vi "Create Datasets.vi"() -> ()   [LabVIEW 2020]
uses:
  ctl/Connection Information.ctl
  <vilib>/addons/database/Connection.llb/Conn ObjectReference.ctl
  <vilib>/addons/database/Connection.llb/DB Tools Open Connec (String).vi
  <vilib>/addons/database/Connection.llb/DB Tools Open Connec (Path).vi
  <vilib>/addons/database/Connection.llb/Conn Execute.vi
  <vilib>/addons/database/Recordset.llb/Rec Fetch Recordset Data (R).vi
  <vilib>/addons/database/Recordset.llb/Rec Destroy - Connection.vi
  <vilib>/addons/database/_DB Variant To Data/Database Variant To Data.xnode
  <vilib>/addons/database/NI_Database_API.lvlib
panel:
  in  "Back Square":bool
  in  "Save Data Set":bool
  in  "Build Query":bool
  out "Query":string
  in  "Records":string[](tree)
  in  "Move Right":bool
  in  "Move Left":bool
  out "error out":errorcluster
  out "data":string[][](array[string])
  out "Get Values on Tree":bool
  in  "Database Tree":string[](tree)
  in  "error in (no error)":errorcluster
  in  "Connect Button":bool
  in  "stop":bool
  in  "Connection Information":T1
  in  "Data Sources":string(combo)
  # "SELECT DATA SOURCE"
  # "SELECT COLUMN"
  # "CREATE DATA SETS"
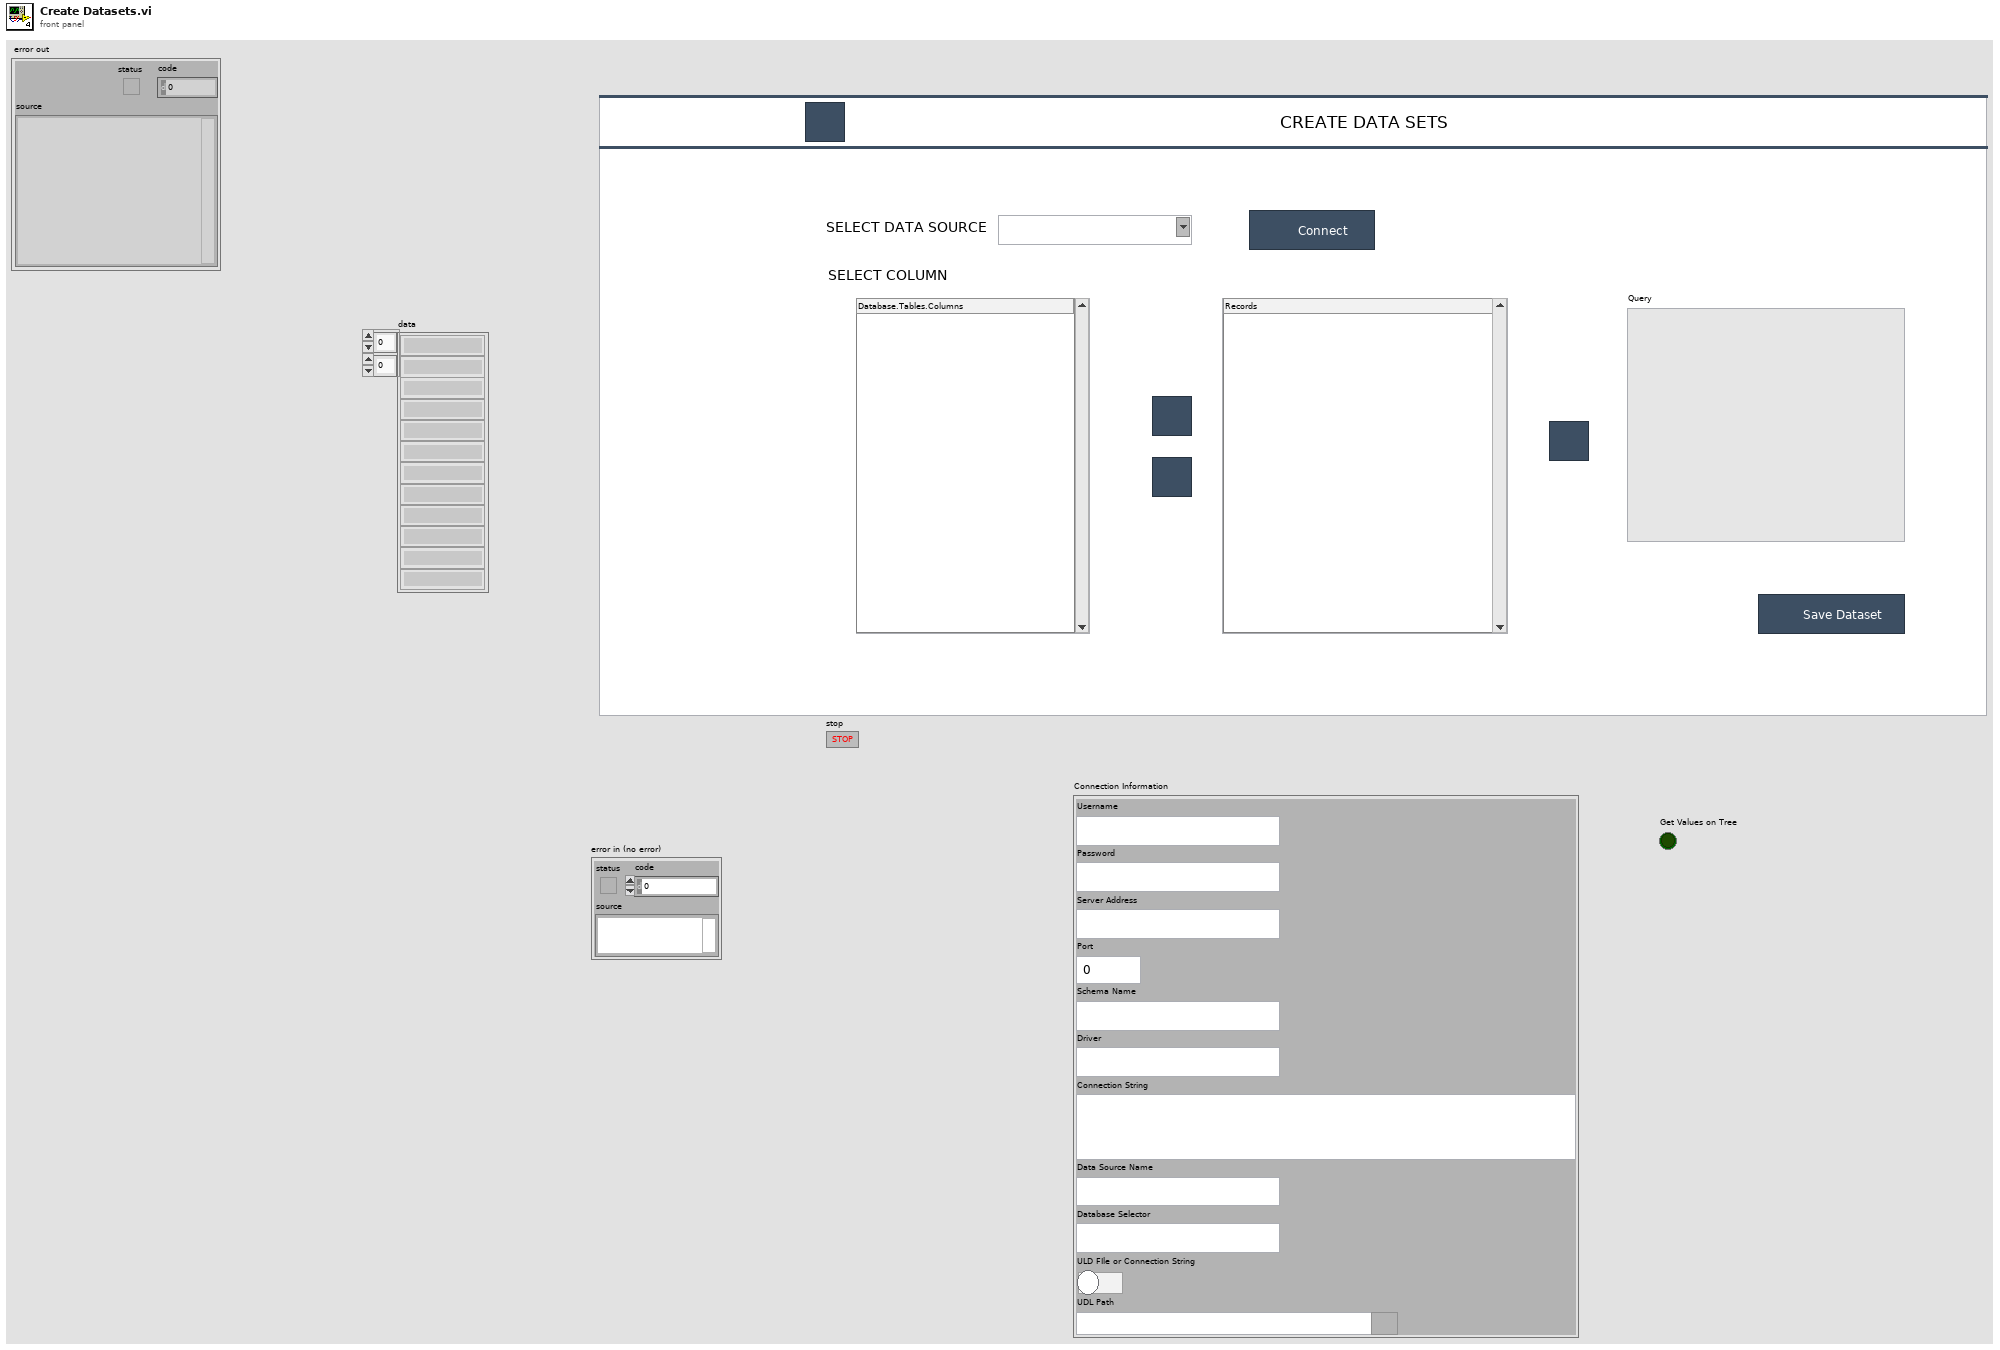
[diagram p1: front panel]
types:
  T1 = typedef "Connection Information.ctl" = cluster{"Username":string, "Password":string, "Server Address":string, "Port":u32, "Schema Name":string, "Driver":string, "Connection String":string, "Data Source Name":string, "Database Selector":string, "ULD FIle or Connection String":bool, "UDL Path":path}
  T2 = typedef "Config Cluster.ctl" = cluster{"MYSQL":cluster{"SHOW DATABASE":string, "SHOW TABLES":string, "SHOW COLUMNS":string}, "SQL Server":cluster{"SHOW DATABASE":string, "SHOW TABLES":string, "SHOW COLUMNS":string}}
  T3 = cluster{"Left Cell String":string, "Child Text":string[], "Child Tag":string, "Item Indent":i32, "Child Only?":bool, "Glyph Index":i32}
  T4 = typedef "NI_Database_API.lvlib/Conn ObjectReference.ctl" = refnum<k1>
  T5 = typedef "NI_Database_API.lvlib/Rec ObjectReference.ctl" = refnum<k1>
  T6 = cluster{"Left Cell String":string, "Child Text":string[], "Child Tag":string, "Item Indent":i32, "Child Only?":bool, "Glyph Index":i32}[]
  T7 = cluster{"Query":string, "DB Type":string, "Data Source name":string}
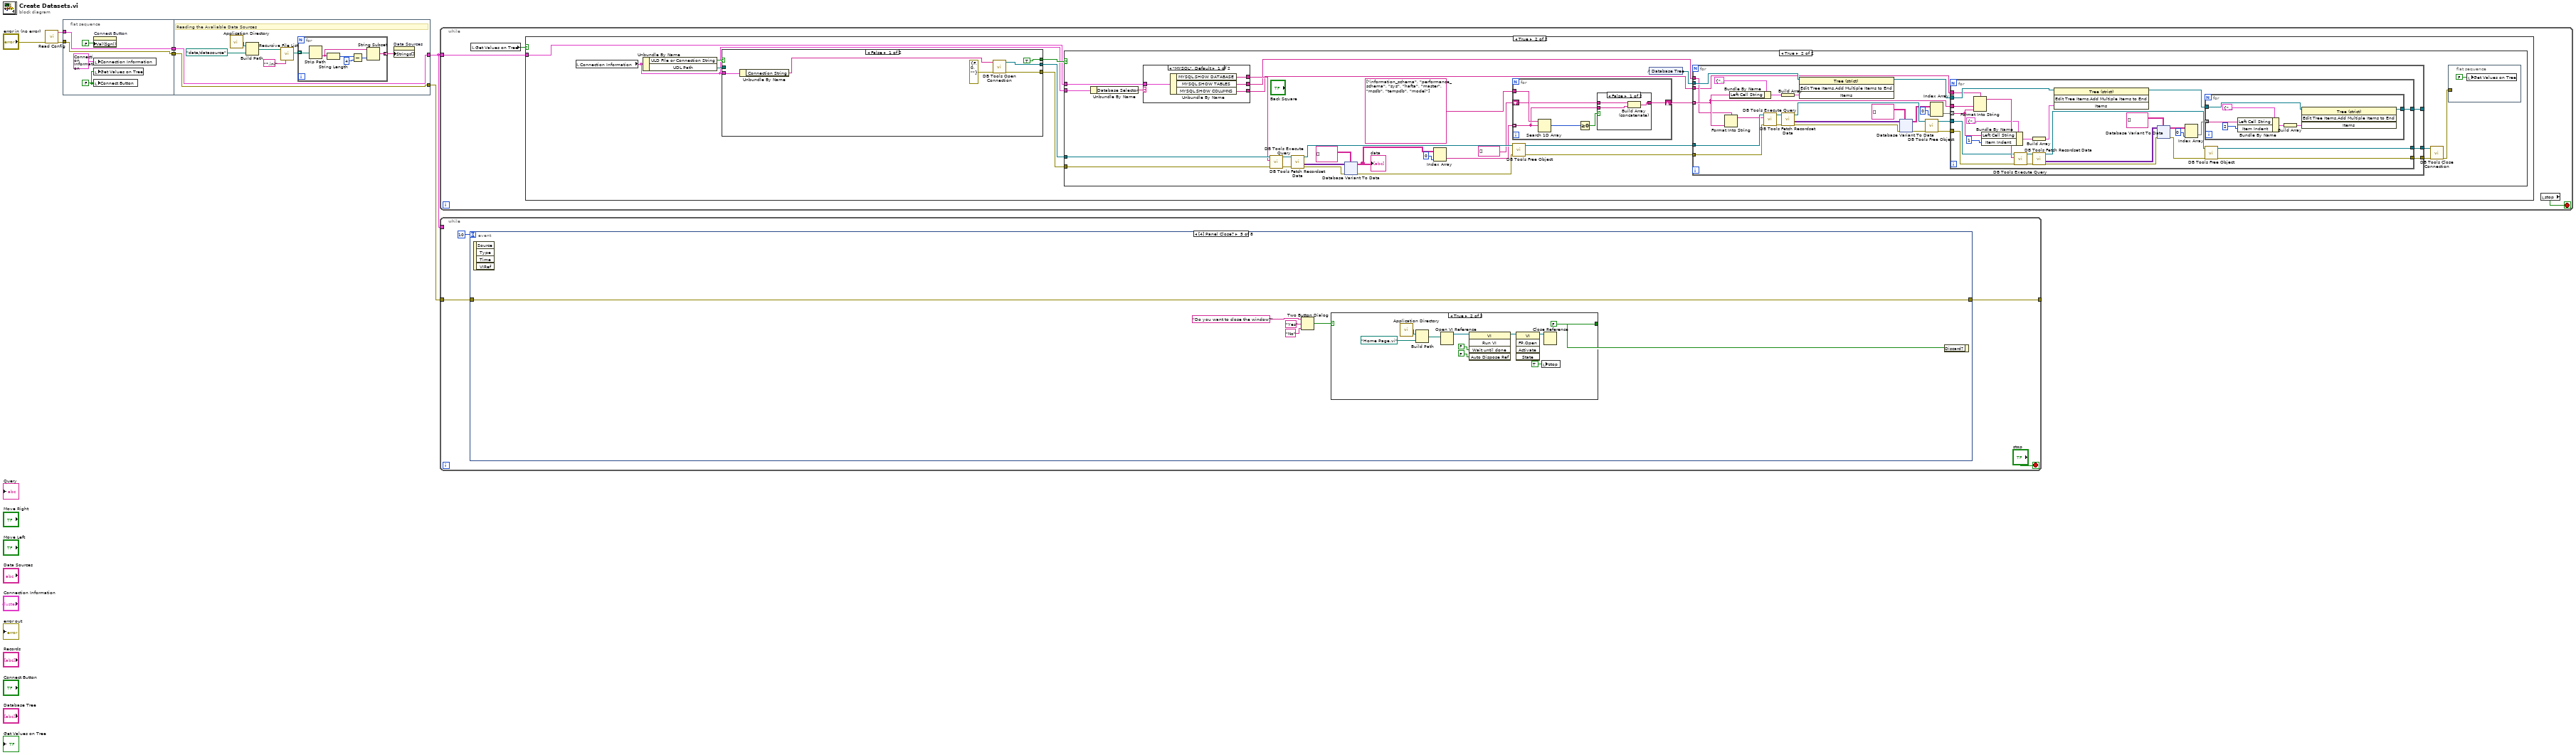
[diagram p0: block diagram]
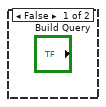
[diagram p2: hidden frame]
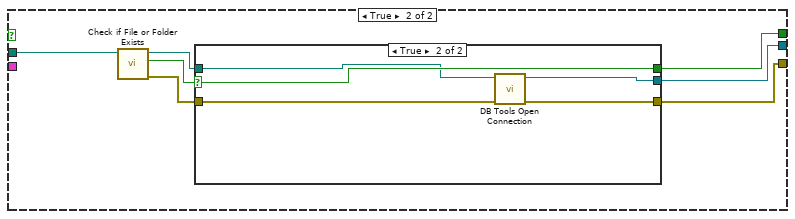
[diagram p3: hidden frame]
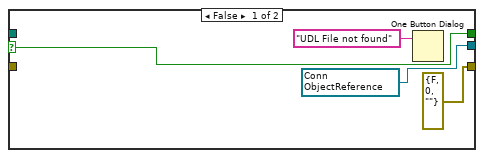
[diagram p4: hidden frame]
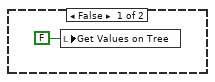
[diagram p5: hidden frame]
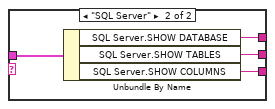
[diagram p6: hidden frame]
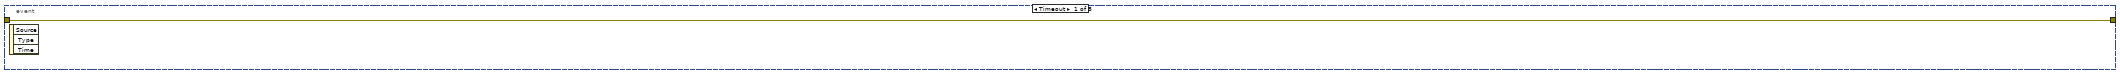
[diagram p8: hidden frame]
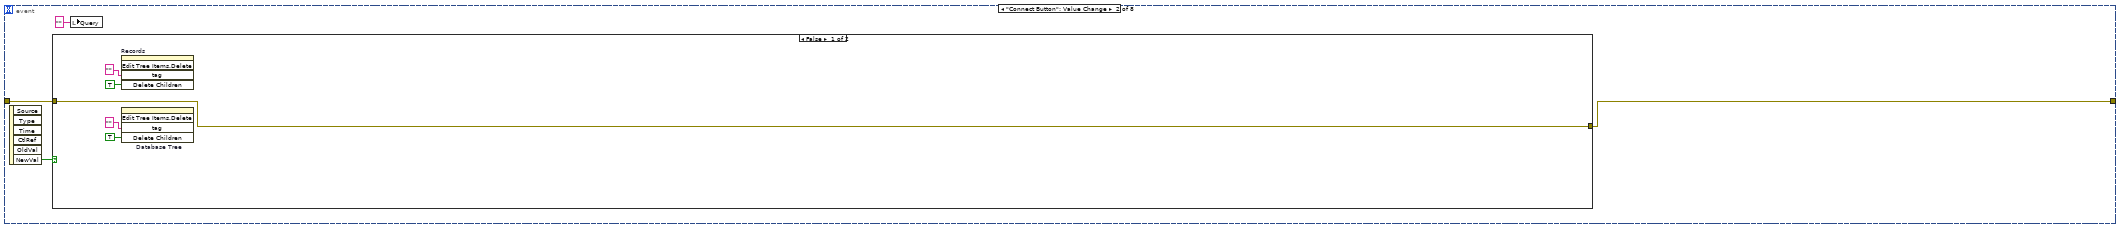
[diagram p9: hidden frame]
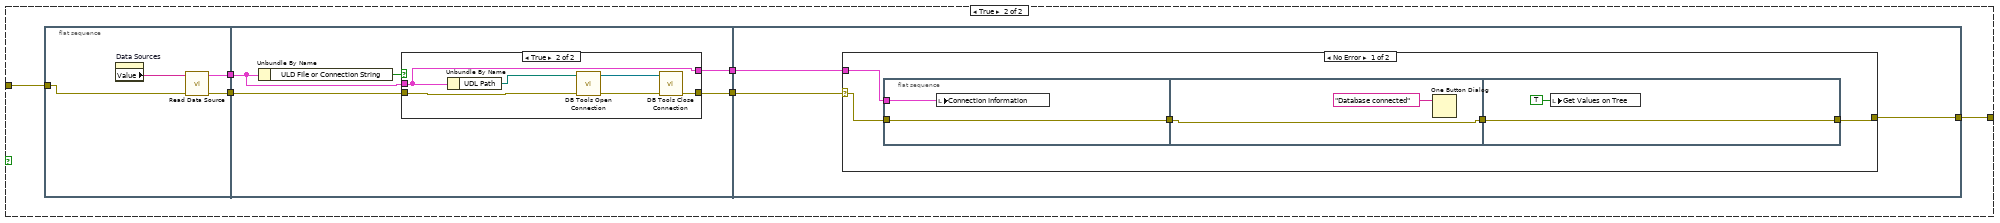
[diagram p10: hidden frame]
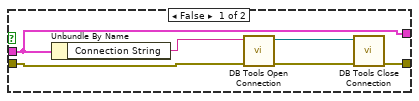
[diagram p11: hidden frame]
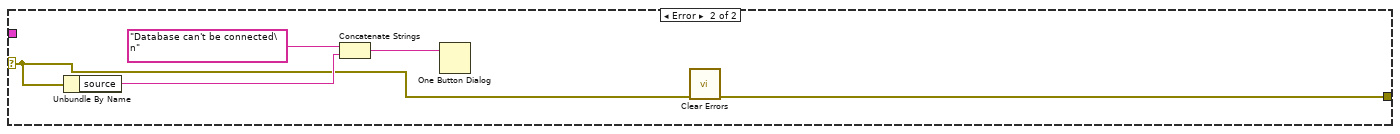
[diagram p12: hidden frame]
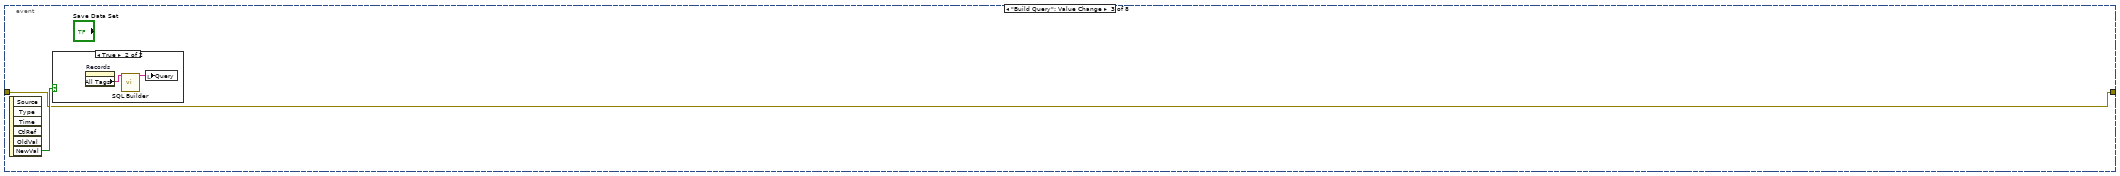
[diagram p13: hidden frame]
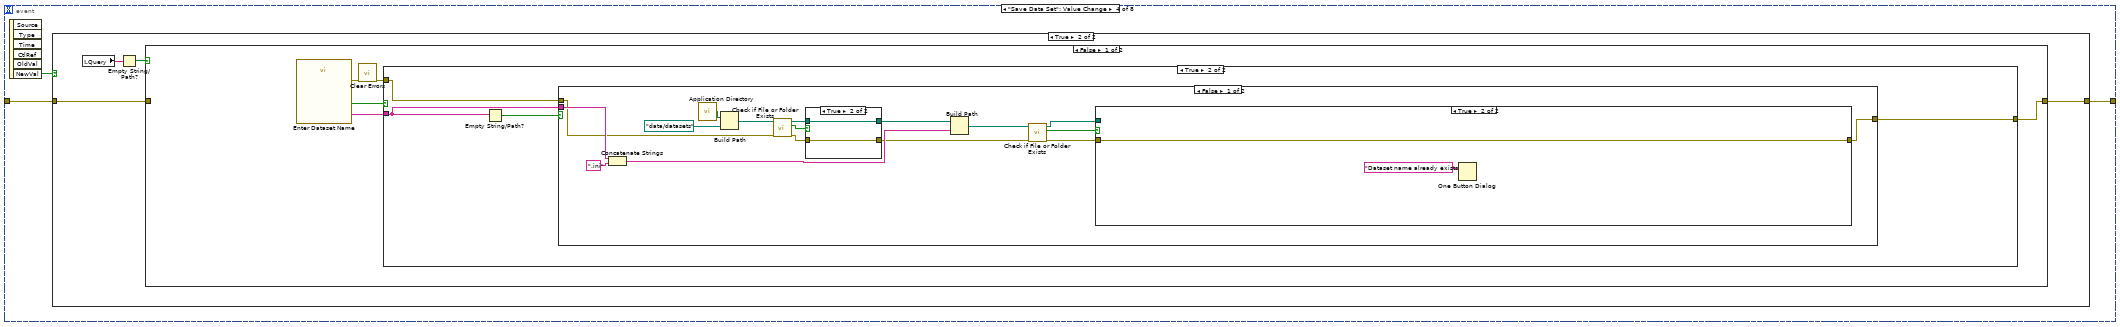
[diagram p15: hidden frame]
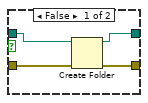
[diagram p18: hidden frame]
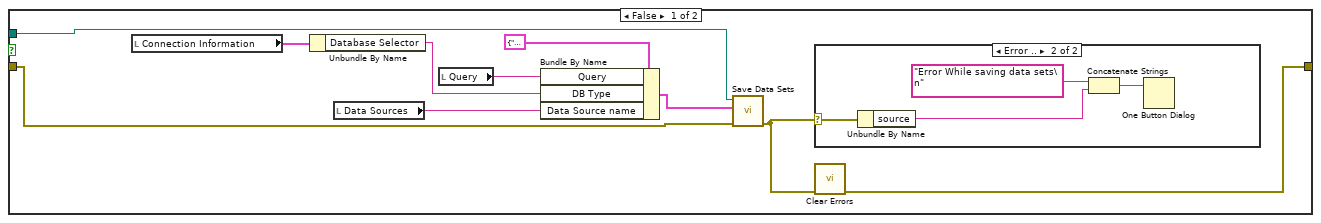
[diagram p19: hidden frame]
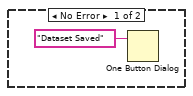
[diagram p20: hidden frame]
diagram:
  n1 = call "Read Config.vi"("error in (no error)"="error in (no error)") -> ("error out"=w1:errorcluster, "Config"=w4:T2)  [unwired: 9 in]
  n2 = flat-sequence {
    tunnel: w1 -> [w12]
    tunnel: [w12] -> w6
    tunnel: [w8] -> w5
    tunnel: w4 -> [w8]
    tunnel: [w20] -> w7
    tunnel: w6 -> [w20]
    tunnel: [w13] -> w3
    tunnel: w5 -> [w13]
    frame #0 {
      w10 = FALSE ("Get Values on Tree")
      n3 = property on="Connect Button" class="Bool (strict)"("Val(Sgnl)"=FALSE ("Value (Signaling)")) -> ()  [unwired: 2 in, 2 out]
      n4 = local write "Connection Information"(T1 {"Username"="", "Password"="", "Server Address"="", "Port"=0, "Schema Name"="", "Driver"="", "Connection String"="", "Data Source Name"="", "Database Selector"="", "ULD FIle or Connection String"=FALSE, "UDL Path"=path ""} ("Connection Information")) -> ()
      n5 = local write "Get Values on Tree"(w10) -> ()
      n6 = local write "Connect Button"(w10) -> ()
    }
    frame #1 {
      # "Reading the Avaliable Data Sources"
      n7 = call <vilib>:"Application Directory.vi"() -> ("Application Directory"=w19:path)
      n8 = Build Path(base path=w19, name or relative path=path "data/datasource") -> (appended path=w17:path)
      n9 = call <vilib>:"Recursive File List.vi"("pattern"="*.ini", "Folder Path"=w17) -> ("All Files in Dir"=w15:path[])  [unwired: 5 in, 4 out]
      n10 = for {
        tunnel: w15 -> [w26] mode=indexing
        tunnel: [w23] -> w14 mode=indexing
        n11 = Strip Path(path=w26) -> (name=w25:string)  [unwired: 1 out]
        n12 = String Length(string=w25) -> (length=w24:i32)
        n13 = Subtract(x=w24, y=4) -> (x-y=w22:i32)
        n14 = String Subset(string=w25, length (rest)=w22) -> (substring=w23:string)  [unwired: 1 in]
      }
      n15 = property on="Data Sources" class="CmbBox"("Strings[]"=w14) -> ()  [unwired: 2 in, 2 out]
    }
  }
  n16 = while {
    tunnel: w3 -> [w28]
    stop <- w29 stop-if-true
    n17 = local read "Get Values on Tree"() -> (w27:bool)
    n18 = case shown="True" w27 {
      tunnel: w28 -> [_ w30]
      frame False {
      }
      frame True {
        n19 = local read "Connection Information"() -> (w31:T1)
        n20 = Unbundle By Name(w31) -> ("ULD FIle or Connection String"=w36:bool, "UDL Path"=w35:path)
        n21 = case shown="False" w36 {
          tunnel: w35 -> [_ w49]
          tunnel: [TRUE ("file or folder exists?") w47] -> w34
          tunnel: [w40 w43] -> w33
          tunnel: [w39 w44] -> w32
          tunnel: w31 -> [w38 _]
          frame False {
            n22 = Unbundle By Name(w38) -> ("Connection String"=w37:string)
            n23 = call-poly <vilib>:"DB Tools Open Connection.vi"("error in (no error)"=errorcluster {"status"=FALSE, "code"=0, "source"=""} ("error out"), "connection information"=w37) -> ("error out"=w40:errorcluster, "connection reference"=w39:T4)  [unwired: 6 in]
          }
          frame True {
            n24 = call <vilib>:"Check if File or Folder Exists.vi"("path"=w49) -> ("error out"=w45:errorcluster, "file or folder exists?"=w48:bool, "dup path"=w46:path)  [unwired: 8 in]
            n25 = case shown="True" w48 {
              selector: w48 -> [w52 w58]
              tunnel: [w52 w58] -> w47
              tunnel: w46 -> [_ w57]
              tunnel: w45 -> [_ w56]
              tunnel: [w51 w55] -> w44
              tunnel: [errorcluster {"status"=FALSE, "code"=0, "source"=""} ("error out") w54] -> w43
              frame False {
                w51 = T4 refnum items=["Connection"] ("connection reference")
                n26 = One Button Dialog(message="UDL File not found") -> ()  [unwired: 1 in, 1 out]
              }
              frame True {
                n27 = call-poly <vilib>:"DB Tools Open Connection.vi"("error in (no error)"=w56, "connection information"=w57) -> ("error out"=w54:errorcluster, "connection reference"=w55:T4)  [unwired: 6 in]
              }
            }
          }
        }
        n28 = case shown="True" w34 {
          tunnel: w31 -> [_ w66]
          tunnel: w33 -> [_ w68]
          tunnel: w32 -> [_ w67]
          tunnel: w30 -> [_ w63]
          frame False {
            n29 = local write "Get Values on Tree"(FALSE ("Get Values on Tree")) -> ()
          }
          frame True {
            n30 = Unbundle By Name(w66) -> ("Database Selector"=w65:string)
            n31 = case shown="\"MYSQL\", Default" w65 {
              tunnel: [w90 w94] -> w64
              tunnel: w63 -> [w91 w95]
              tunnel: [w89 w93] -> w62
              tunnel: [w88 w92] -> w61
              frame "MYSQL", Default {
                n32 = Unbundle By Name(w91) -> ("MYSQL.SHOW DATABASE"=w90:string, "MYSQL.SHOW TABLES"=w89:string, "MYSQL.SHOW COLUMNS"=w88:string)
              }
              frame "SQL Server" {
                n33 = Unbundle By Name(w95) -> ("SQL Server.SHOW DATABASE"=w94:string, "SQL Server.SHOW TABLES"=w93:string, "SQL Server.SHOW COLUMNS"=w92:string)
              }
            }
            n34 = call-poly <vilib>:"DB Tools Execute Query.vi"("error in (no error)"=w68, "SQL query"=w64, "connection reference"=w67) -> ("error out"=w85:errorcluster, "recordset reference"=w86:T5)  [unwired: 5 in]
            n35 = call-poly <vilib>:"DB Tools Fetch Recordset Data.vi"("error in (no error)"=w85, "recordset reference"=w86) -> ("error out"=w81:errorcluster, "recordset data"=w83:variant[][], "recordset reference out"=w84:T5)  [unwired: 3 in]
            n36 = xnode "Database Variant To Data"("database variant"=w83, "error in (no error)"=w81, "type"=string[][] []) -> ("data"=w79:string[][], "error out"=w80:errorcluster)
            "data" <- w79
            n37 = Index Array(array=w79, index (col)=0 ("disabled index (col)")) -> (element=w71:string[])  [unwired: 1 in]
            n38 = for {
              tunnel: w71 -> [w96] mode=indexing
              shift-right: [w98] -> w70
              shift-left: string[] [] -> [w97]
              tunnel: string[] ["information_schema", "performance_schema", "sys", "hafta", "master", "msdb", "tempdb", "model"] -> [w101]
              n39 = Search 1D Array(1D array=w101, element=w96) -> (index of element=w100:i32)  [unwired: 1 in]
              n40 = Greater Or Equal To 0?(x=w100) -> (x >= 0?=w99:bool)
              n41 = case shown="False" w99 {
                tunnel: [w102 w105] -> w98
                tunnel: w97 -> [w103 w105]
                tunnel: w96 -> [w104 _]
                frame False {
                  n42 = Build Array (concatenate)(w103, w104) -> (w102:string[])
                }
                frame True {
                }
              }
            }
            n43 = call-poly <vilib>:"DB Tools Free Object.vi"("error in (no error)"=w80, "recordset reference"=w84) -> ("error out"=w76:errorcluster, "connection reference"=w77:T4)  [unwired: 8 in]
            n44 = control-ref of="Database Tree"() -> (w69:refnum<vi>)
            n45 = for {
              tunnel: w77 -> [w130]
              tunnel: w76 -> [w129]
              tunnel: w69 -> [w131]
              tunnel: w70 -> [w109] mode=indexing
              tunnel: [w115] -> w75
              tunnel: [w114] -> w74
              tunnel: [w108] -> _
              tunnel: w62 -> [w107]
              tunnel: w61 -> [w106]
              n46 = Format Into String(format string=w107, w109) -> (resulting string=w128:string)  [unwired: 2 in, 1 out]
              n47 = Bundle By Name(cluster=T3 {"Left Cell String"="", "Child Text"=[], "Child Tag"="", "Item Indent"=0, "Child Only?"=FALSE, "Glyph Index"=0} ("Item"), "Left Cell String"=w109) -> (w112:T3)
              n48 = call-poly <vilib>:"DB Tools Execute Query.vi"("error in (no error)"=w129, "SQL query"=w128, "connection reference"=w130) -> ("error out"=w126:errorcluster, "recordset reference"=w127:T5)  [unwired: 5 in]
              n49 = Build Array(w112) -> (w111:T6)
              n50 = call-poly <vilib>:"DB Tools Fetch Recordset Data.vi"("error in (no error)"=w126, "recordset reference"=w127) -> ("error out"=w122:errorcluster, "recordset data"=w123:variant[][], "recordset reference out"=w125:T5)  [unwired: 3 in]
              n51 = invoke on="Invoke Node" class="Tree (strict)" method="Edit Tree Items.Add Multiple Items to End"(reference=w131, "Items"=w111) -> (reference out=w110:refnum<vi>)  [unwired: 2 in, 3 out]
              n52 = xnode "Database Variant To Data"("database variant"=w123, "error in (no error)"=w122, "type"=string[][] []) -> ("data"=w120:string[][], "error out"=w121:errorcluster)
              n53 = call-poly <vilib>:"DB Tools Free Object.vi"("error in (no error)"=w121, "recordset reference"=w125) -> ("error out"=w116:errorcluster, "connection reference"=w117:T4)  [unwired: 8 in]
              n54 = Index Array(array=w120, index (col)=0 ("disabled index (col)")) -> (element=w118:string[])  [unwired: 1 in]
              n55 = for {
                tunnel: w118 -> [w177] mode=indexing
                tunnel: w117 -> [w190]
                tunnel: w116 -> [w189]
                tunnel: [w188] -> w115
                tunnel: [w187] -> w114
                tunnel: w110 -> [w181]
                tunnel: w109 -> [w178]
                tunnel: [w179] -> w108
                tunnel: w106 -> [w176]
                n56 = Format Into String(format string=w176, w178, w177) -> (resulting string=w191:string)  [unwired: 2 in, 1 out]
                n57 = Bundle By Name(cluster=T3 {"Left Cell String"="", "Child Text"=[], "Child Tag"="", "Item Indent"=0, "Child Only?"=FALSE, "Glyph Index"=0} ("Item"), "Left Cell String"=w177, "Item Indent"=1) -> (w186:T3)
                n58 = call-poly <vilib>:"DB Tools Execute Query.vi"("error in (no error)"=w189, "SQL query"=w191, "connection reference"=w190) -> ("error out"=w193:errorcluster, "recordset reference"=w192:T5)  [unwired: 5 in]
                n59 = Build Array(w186) -> (w184:T6)
                n60 = call-poly <vilib>:"DB Tools Fetch Recordset Data.vi"("error in (no error)"=w193, "recordset reference"=w192) -> ("error out"=w197:errorcluster, "recordset data"=w196:variant[][], "recordset reference out"=w194:T5)  [unwired: 3 in]
                n61 = invoke on="Invoke Node" class="Tree (strict)" method="Edit Tree Items.Add Multiple Items to End"(reference=w181, "Items"=w184) -> (reference out=w180:refnum<vi>)  [unwired: 2 in, 3 out]
                n62 = xnode "Database Variant To Data"("database variant"=w196, "error in (no error)"=w197, "type"=string[][] []) -> ("data"=w199:string[][], "error out"=w198:errorcluster)
                n63 = Index Array(array=w199, index (col)=0 ("disabled index (col)")) -> (element=w182:string[])  [unwired: 1 in]
                n64 = for {
                  tunnel: w182 -> [w203] mode=indexing
                  tunnel: w180 -> [w202]
                  tunnel: [w201] -> w179
                  n65 = Bundle By Name(cluster=T3 {"Left Cell String"="", "Child Text"=[], "Child Tag"="", "Item Indent"=0, "Child Only?"=FALSE, "Glyph Index"=0} ("Item"), "Left Cell String"=w203, "Item Indent"=2) -> (w204:T3)
                  n66 = Build Array(w204) -> (w206:T6)
                  n67 = invoke on="Invoke Node" class="Tree (strict)" method="Edit Tree Items.Add Multiple Items to End"(reference=w202, "Items"=w206) -> (reference out=w201:refnum<vi>)  [unwired: 2 in, 3 out]
                }
                n68 = call-poly <vilib>:"DB Tools Free Object.vi"("error in (no error)"=w198, "recordset reference"=w194) -> ("error out"=w188:errorcluster, "connection reference"=w187:T4)  [unwired: 8 in]
              }
            }
            n69 = call <vilib>:"DB Tools Close Connection.vi"("error in (no error)"=w75, "connection reference"=w74) -> ("error out"=w60:errorcluster)  [unwired: 5 in]
            n70 = flat-sequence {
              tunnel: w60 -> [_]
              frame #0 {
                n71 = local write "Get Values on Tree"(FALSE ("Get Values on Tree")) -> ()
              }
            }
          }
        }
      }
    }
    n72 = local read "stop"() -> (w29:bool)
  }
  n73 = while {
    tunnel: w7 -> [w297]
    tunnel: w3 -> [_]
    tunnel: [w296] -> _
    stop <- "stop" stop-if-true
    n74 = event shown="[4] Panel Close?" {
      selector: _ -> [_ _ _ _ _ _ _ _]
      dyn-events: _ -> [_ _ _ _ _ _ _ _]
      timeout: 10 -> [_ _ _ _ _ _ _ _]
      tunnel: w297 -> [w300 w303 w356 w360 w424 _ w453 w515]
      tunnel: [w300 w302 w356 w361 w424 _ w453 w515] -> w296
      event Timeout {
        n75 = event-data() -> ()  [unwired: 1 in, 3 out]
      }
      event "Connect Button": Value Change {
        n76 = event-data() -> ("NewVal"=w304:bool)  [unwired: 1 in, 5 out]
        n77 = case shown="False" w304 {
          tunnel: w303 -> [w309 w312]
          tunnel: [w309 w311] -> w302
          frame False {
            n78 = invoke on="Records" class="Tree (strict)" method="Edit Tree Items.Delete"("tag"="" ("Tag"), "Delete Children"=TRUE ("Delete Children?")) -> ()  [unwired: 3 in, 5 out]
            n79 = invoke on="Database Tree" class="Tree (strict)" method="Edit Tree Items.Delete"("tag"="" ("Tag"), "Delete Children"=TRUE ("Delete Children?")) -> ()  [unwired: 3 in, 5 out]
          }
          frame True {
            n80 = flat-sequence {
              tunnel: [w318] -> w315
              tunnel: [w317] -> w314
              tunnel: w312 -> [w316]
              tunnel: w315 -> [w324]
              tunnel: w314 -> [w321]
              tunnel: [w323] -> w313
              tunnel: [w320] -> w310
              tunnel: w313 -> [w339]
              tunnel: [w337] -> w311
              tunnel: w310 -> [w338]
              frame #0 {
                n81 = property on="Data Sources" class="CmbBox"() -> ("Value"=w319:string)  [unwired: 2 in, 2 out]
                n82 = call "Read Data Source.vi"("error in (no error)"=w316, "Data Source Name"=w319) -> ("error out"=w318:errorcluster, "Connection Information"=w317:T1)  [unwired: 8 in]
              }
              frame #1 {
                n83 = Unbundle By Name(w321) -> ("ULD FIle or Connection String"=w322:bool)
                n84 = case shown="True" w322 {
                  tunnel: w324 -> [w327 w334]
                  tunnel: [w326 w333] -> w323
                  tunnel: w321 -> [w325 w331]
                  tunnel: [w325 w331] -> w320
                  frame False {
                    n85 = Unbundle By Name(w325) -> ("Connection String"=w328:string)
                    n86 = call-poly <vilib>:"DB Tools Open Connection.vi"("error in (no error)"=w327, "connection information"=w328) -> ("error out"=w330:errorcluster, "connection reference"=w329:T4)  [unwired: 6 in]
                    n87 = call <vilib>:"DB Tools Close Connection.vi"("error in (no error)"=w330, "connection reference"=w329) -> ("error out"=w326:errorcluster)  [unwired: 5 in]
                  }
                  frame True {
                    n88 = Unbundle By Name(w331) -> ("UDL Path"=w332:path)
                    n89 = call-poly <vilib>:"DB Tools Open Connection.vi"("error in (no error)"=w334, "connection information"=w332) -> ("error out"=w336:errorcluster, "connection reference"=w335:T4)  [unwired: 6 in]
                    n90 = call <vilib>:"DB Tools Close Connection.vi"("error in (no error)"=w336, "connection reference"=w335) -> ("error out"=w333:errorcluster)  [unwired: 5 in]
                  }
                }
              }
              frame #2 {
                n91 = case shown="No Error" w339 {
                  selector: w339 -> [w340 w352]
                  tunnel: w338 -> [w344 _]
                  tunnel: [w343 w351] -> w337
                  frame No Error {
                    n92 = flat-sequence {
                      tunnel: w344 -> [w346]
                      tunnel: [w345] -> w341
                      tunnel: w340 -> [w345]
                      tunnel: [w347] -> w342
                      tunnel: w341 -> [w347]
                      tunnel: [w349] -> w343
                      tunnel: w342 -> [w349]
                      frame #0 {
                        n93 = local write "Connection Information"(w346) -> ()
                      }
                      frame #1 {
                        n94 = One Button Dialog(message="Database connected") -> ()  [unwired: 1 in, 1 out]
                      }
                      frame #2 {
                        n95 = local write "Get Values on Tree"(TRUE ("Get Values on Tree")) -> ()
                      }
                    }
                  }
                  frame Error {
                    n96 = Unbundle By Name(w352) -> ("source"=w354:string)
                    n97 = Concatenate Strings("Database can't be connected\n" ("message"), w354) -> (w353:string)
                    n98 = One Button Dialog(message=w353) -> ()  [unwired: 1 in, 1 out]
                    n99 = call <vilib>:"Clear Errors.vi"("error in (no error)"=w352) -> ("error out"=w351:errorcluster)  [unwired: 5 in, 1 out]
                  }
                }
              }
            }
          }
        }
        n100 = local write "Query"("" ("Query")) -> ()
      }
      event "Build Query": Value Change {
        n101 = event-data() -> ("NewVal"=w357:bool)  [unwired: 1 in, 5 out]
        n102 = case shown="True" w357 {
          frame False {
          }
          frame True {
            n103 = property on="Records" class="Tree (strict)"() -> ("All Tags"=w358:string[])  [unwired: 2 in, 2 out]
            n104 = call "SQL Builder.vi"("SELECTED COLUMNS"=w358) -> ("Built Query"=w359:string)  [unwired: 10 in]
            n105 = local write "Query"(w359) -> ()
          }
        }
      }
      event "Save Data Set": Value Change {
        n106 = event-data() -> ("NewVal"=w362:bool)  [unwired: 1 in, 5 out]
        n107 = case shown="True" w362 {
          tunnel: [w363 w365] -> w361
          tunnel: w360 -> [w363 w364]
          frame False {
          }
          frame True {
            n108 = local read "Query"() -> (w367:string)
            n109 = Empty String/Path?(string/path=w367) -> (empty?=w366:bool)
            n110 = case shown="False" w366 {
              tunnel: [w368 w421] -> w365
              tunnel: w364 -> [_ w421]
              frame False {
                n111 = call "Enter Dataset Name"() -> ("Dataset Name"=w369:string, "OK"=w372:bool, "error out"=w371:errorcluster)  [unwired: 17 in]
                n112 = call <vilib>:"Clear Errors.vi"("error in (no error)"=w371) -> ("error out"=w370:errorcluster)  [unwired: 5 in, 1 out]
                n113 = case shown="True" w372 {
                  tunnel: w370 -> [w373 w375]
                  tunnel: w369 -> [_ w376]
                  tunnel: [w373 w374] -> w368
                  frame False {
                  }
                  frame True {
                    n114 = Empty String/Path?(string/path=w376) -> (empty?=w377:bool)
                    n115 = case shown="False" w377 {
                      tunnel: w376 -> [w394 _]
                      tunnel: w375 -> [w385 w418]
                      tunnel: [w378 w418] -> w374
                      frame False {
                        n116 = Concatenate Strings(w394, ".ini" ("string")) -> (w392:string)
                        n117 = call <vilib>:"Application Directory.vi"() -> ("Application Directory"=w391:path)
                        n118 = Build Path(base path=w391, name or relative path=path "data/datasets") -> (appended path=w384:path)
                        n119 = call <vilib>:"Check if File or Folder Exists.vi"("error in (no error)"=w385, "path"=w384) -> ("error out"=w379:errorcluster, "file or folder exists?"=w383:bool, "dup path"=w382:path)  [unwired: 7 in]
                        n120 = case shown="True" w383 {
                          tunnel: w382 -> [w398 w400]
                          tunnel: [w397 w400] -> w381
                          tunnel: [w396 w399] -> w380
                          tunnel: w379 -> [w395 w399]
                          frame False {
                            n121 = Create Folder(path (use dialog)=w398, error in=w395) -> (created path=w397:path, error out=w396:errorcluster)  [unwired: 1 in, 1 out]
                          }
                          frame True {
                          }
                        }
                        n122 = Build Path(base path=w381, name or relative path=w392) -> (appended path=w389:path)
                        n123 = call <vilib>:"Check if File or Folder Exists.vi"("error in (no error)"=w380, "path"=w389) -> ("error out"=w386:errorcluster, "file or folder exists?"=w387:bool, "dup path"=w388:path)  [unwired: 7 in]
                        n124 = case shown="True" w387 {
                          tunnel: w388 -> [w410 _]
                          tunnel: w386 -> [w409 w417]
                          tunnel: [w401 w417] -> w378
                          frame False {
                            n125 = local read "Connection Information"() -> (w404:T1)
                            n126 = Unbundle By Name(w404) -> ("Database Selector"=w403:string)
                            n127 = local read "Data Sources"() -> (w406:string)
                            n128 = local read "Query"() -> (w405:string)
                            n129 = Bundle By Name(cluster=T7 {"Query"="", "DB Type"="", "Data Source name"=""} ("Information"), "Query"=w405, "DB Type"=w403, "Data Source name"=w406) -> (w407:T7)
                            n130 = call "Save Data Sets.vi"("error in (no error)"=w409, "Information"=w407, "Saving Path"=w410) -> ("error out"=w402:errorcluster)  [unwired: 8 in]
                            n131 = case shown="Error .." w402 {
                              selector: w402 -> [_ w415]
                              frame No Error {
                                n132 = One Button Dialog(message="Dataset Saved") -> ()  [unwired: 1 in, 1 out]
                              }
                              frame Error {
                                n133 = Unbundle By Name(w415) -> ("source"=w413:string)
                                n134 = Concatenate Strings("Error While saving data sets\n" ("message"), w413) -> (w412:string)
                                n135 = One Button Dialog(message=w412) -> ()  [unwired: 1 in, 1 out]
                              }
                            }
                            n136 = call <vilib>:"Clear Errors.vi"("error in (no error)"=w402) -> ("error out"=w401:errorcluster)  [unwired: 5 in, 1 out]
                          }
                          frame True {
                            n137 = One Button Dialog(message="Dataset name already exists") -> ()  [unwired: 1 in, 1 out]
                          }
                        }
                      }
                      frame True {
                        n138 = One Button Dialog(message="Enter Valid dataset name", button name ("OK")="OK") -> ()  [unwired: 1 out]
                      }
                    }
                  }
                }
              }
              frame True {
                n139 = One Button Dialog(message="Build Query Before Saving", button name ("OK")="OK") -> ()  [unwired: 1 out]
              }
            }
          }
        }
      }
      event Panel Close? {
        n140 = event-data() -> ()  [unwired: 1 in, 4 out]
        n141 = Two Button Dialog(message="Do you want to close the window?", 1:"No" ("F button name (\"Cancel\")"), 2:"Yes" ("T button name (\"OK\")")) -> (T button?=w426:bool)
        n142 = case shown="True" w426 {
          tunnel: [TRUE ("Discard?") FALSE ("Discard?")] -> w425
          frame False {
          }
          frame True {
            n143 = call <vilib>:"Application Directory.vi"() -> ("Application Directory"=w439:path)
            n144 = Build Path(base path=w439, name or relative path=path "Home Page.vi") -> (appended path=w437:path)
            n145 = Open VI Reference(vi path=w437) -> (vi reference=w436:refnum<vi>)  [unwired: 5 in, 1 out]
            n146 = invoke class="VI" method="Run VI"(reference=w436, "Wait until done"=FALSE ("Wait Until Done"), "Auto Dispose Ref"=FALSE ("Auto Dispose Reference")) -> (reference out=w435:refnum<vi>)  [unwired: 2 in, 4 out]
            n147 = invoke class="VI" method="FP.Open"(reference=w435) -> (reference out=w432:refnum<vi>)  [unwired: 4 in, 4 out]
            n148 = local write "stop"(TRUE ("stop")) -> ()
            n149 = Close Reference(reference=w432) -> ()  [unwired: 1 in, 1 out]
          }
        }
        n150 = event-data("Discard?"=w425) -> ()  [unwired: 1 in, 1 out]
      }
      event "Back Square": Value Change {
        n151 = event-data() -> ("NewVal"=w441:bool)  [unwired: 1 in, 5 out]
        n152 = case shown="True" w441 {
          frame False {
          }
          frame True {
            n153 = call <vilib>:"Application Directory.vi"() -> ("Application Directory"=w450:path)
            n154 = Build Path(base path=w450, name or relative path=path "Home Page.vi") -> (appended path=w449:path)
            n155 = Open VI Reference(vi path=w449) -> (vi reference=w448:refnum<vi>)  [unwired: 5 in, 1 out]
            n156 = invoke class="VI" method="Run VI"(reference=w448, "Wait until done"=FALSE ("Wait Until Done"), "Auto Dispose Ref"=FALSE ("Auto Dispose Reference")) -> (reference out=w447:refnum<vi>)  [unwired: 2 in, 4 out]
            n157 = invoke class="VI" method="FP.Open"(reference=w447) -> (reference out=w446:refnum<vi>)  [unwired: 4 in, 4 out]
            n158 = Close Reference(reference=w446) -> (error out=w442:errorcluster)  [unwired: 1 in]
            n159 = flat-sequence {
              tunnel: w442 -> [_]
              frame #0 {
                n160 = control-ref of="This VI"() -> (w452:refnum<vi>)
                n161 = local write "stop"(TRUE ("stop")) -> ()
                n162 = invoke class="VI" method="FP.Close"(reference=w452) -> ()  [unwired: 2 in, 3 out]
              }
            }
          }
        }
      }
      event "Move Right": Value Change {
        n163 = event-data() -> ("NewVal"=w455:bool)  [unwired: 1 in, 5 out]
        n164 = case shown="True" w455 {
          frame False {
          }
          frame True {
            n165 = local read "Database Tree"() -> (w465:string[])
            n166 = Index Array(array=w465, index=0) -> (element=w464:string)
            n167 = Empty String/Path?(string/path=w464) -> (empty?=w466:bool)
            n168 = case shown="False" w466 {
              tunnel: w464 -> [w486 _]
              tunnel: [w492 "" ("Navigate Tree:Get Parent")] -> w456
              tunnel: [w489 "" ("Navigate Tree:Get Parent")] -> w457
              tunnel: [w488 ""] -> w458
              frame False {
                n169 = control-ref of="Database Tree"() -> (w487:refnum<vi>)
                n170 = invoke class="Tree (strict)" method="Navigate Tree.Get Parent"(reference=w487, "tag"=w486) -> (reference out=w493:refnum<vi>, "Navigate Tree:Get Parent"=w491:string)  [unwired: 2 in, 2 out]
                n171 = Empty String/Path?(string/path=w491) -> (empty?=w490:bool)
                n172 = case shown="False" w490 {
                  tunnel: w493 -> [w501 _]
                  tunnel: [w498 w511] -> w492
                  tunnel: w491 -> [w497 _]
                  tunnel: [w496 "" ("Navigate Tree:Get Parent")] -> w489
                  tunnel: w486 -> [w494 w511]
                  tunnel: [w494 ""] -> _
                  tunnel: [w495 ""] -> w488
                  frame False {
                    n173 = invoke class="Tree (strict)" method="Navigate Tree.Get Parent"(reference=w501, "tag"=w497) -> ("Navigate Tree:Get Parent"=w499:string)  [unwired: 2 in, 3 out]
                    n174 = Empty String/Path?(string/path=w499) -> (empty?=w500:bool)
                    n175 = case shown="False" w500 {
                      tunnel: w499 -> [w504 _]
                      tunnel: [w504 w507] -> w498
                      tunnel: w497 -> [w503 w507]
                      tunnel: [w503 w506] -> w496
                      tunnel: w494 -> [w502 w506]
                      tunnel: [w502 ""] -> w495
                      frame False {
                      }
                      frame True {
                      }
                    }
                  }
                  frame True {
                  }
                }
              }
              frame True {
              }
            }
            n176 = Empty String/Path?(string/path=w458) -> (empty?=w460:bool)
            n177 = Empty String/Path?(string/path=w456) -> (empty?=w462:bool)
            n178 = Empty String/Path?(string/path=w457) -> (empty?=w461:bool)
            n179 = Compound Arithmetic op=OR(w462, w461, w460) -> (w459:bool)
            n180 = case shown="False" w459 {
              tunnel: w458 -> [w467 _]
              tunnel: w457 -> [w477 _]
              tunnel: w456 -> [w475 _]
              frame False {
                n181 = call "Remove Tree Underscore.vi"("Input String"=w467) -> ("Data"=w468:string)  [unwired: 1 out]
                n182 = control-ref of="Records"() -> (w471:refnum<vi>)
                n183 = property class="Tree (strict)"(reference=w471) -> (reference out=w470:refnum<vi>, "All Tags"=w469:string[])  [unwired: 1 in, 1 out]
                n184 = Concatenate Strings(w475, "." ("string"), w477, "." ("string"), w468) -> (w472:string)
                n185 = Search 1D Array(1D array=w469, element=w472) -> (index of element=w474:i32)  [unwired: 1 in]
                n186 = Greater Or Equal To 0?(x=w474) -> (x >= 0?=w473:bool)
                n187 = case shown="False" w473 {
                  tunnel: w472 -> [w481 _]
                  tunnel: w470 -> [w483 _]
                  frame False {
                    n188 = Bundle By Name(cluster=T3 {"Left Cell String"="", "Child Text"=[], "Child Tag"="", "Item Indent"=0, "Child Only?"=FALSE, "Glyph Index"=0} ("Item"), "Left Cell String"=w481) -> (w480:T3)
                    n189 = Build Array(w480) -> (w479:T6)
                    n190 = invoke on="Invoke Node" class="Tree (strict)" method="Edit Tree Items.Add Multiple Items to End"(reference=w483, "Items"=w479) -> ()  [unwired: 2 in, 4 out]
                  }
                  frame True {
                    n191 = One Button Dialog(message="Selected column\nis already exists") -> ()  [unwired: 1 in, 1 out]
                  }
                }
              }
              frame True {
                n192 = One Button Dialog(message="Select only columns") -> ()  [unwired: 1 in, 1 out]
              }
            }
          }
        }
        n193 = local write "Query"("" ("Query")) -> ()
      }
      event "Move Left": Value Change {
        n194 = event-data() -> ("NewVal"=w517:bool)  [unwired: 1 in, 5 out]
        n195 = case shown="True" w517 {
          frame False {
          }
          frame True {
            n196 = local read "Records"() -> (w521:string[])
            n197 = Index Array(array=w521, index=0) -> (element=w520:string)
            n198 = control-ref of="Records"() -> (w518:refnum<vi>)
            n199 = Empty String/Path?(string/path=w520) -> (empty?=w522:bool)
            n200 = case shown="False" w522 {
              tunnel: w520 -> [w524 _]
              tunnel: w518 -> [w525 _]
              frame False {
                n201 = invoke class="Tree (strict)" method="Edit Tree Items.Delete"(reference=w525, "tag"=w524, "Delete Children"=TRUE ("Delete Children?")) -> ()  [unwired: 2 in, 5 out]
              }
              frame True {
                (unwired) ""
                (unwired) "" ("Navigate Tree:Get Parent")
                (unwired) "" ("Navigate Tree:Get Parent")
              }
            }
          }
        }
        n202 = local write "Query"("" ("Query")) -> ()
      }
    }
  }
